vi "Wait For Debounce External Relays.vi"(11 "error in":errorcluster, 13 "Wait (ms)":u32=5) -> (15 "error out":errorcluster)   [LabVIEW 2021, in "DMM_Scan PXI RLY Driver 32V-16C.lvlib"]
doc: "Debounce wait time based on the external relay timing specification. Typical default value is 5 ms, but needs to be adjusted based on the specific selection of external relay used. \n\nIncorrect values (too short) will affect the accuracy of the measurements."
uses:
  DMM_Scan PXI RLY Driver 32V-16C.lvlib
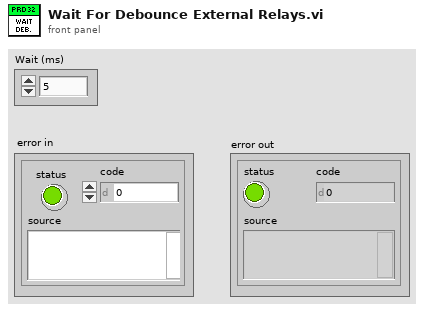
[diagram p1: front panel]
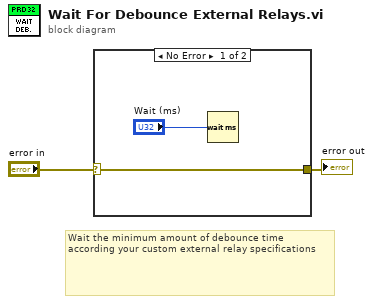
[diagram p0: block diagram]
diagram:
  # "Wait the minimum amount of debounce time according your custom external relay specifications"
  n1 = case shown="No Error" "error in" {
    selector: "error in" -> [w4 w5]
    tunnel: [w4 w5] -> w1
    frame No Error {
      n2 = Wait (ms)(milliseconds to wait="Wait (ms)") -> ()  [unwired: 1 out]
    }
    frame Error {
    }
  }
  "error out" <- w1
